vi "String_Find Any Expresion.vi"(5 "Multiline? (F)":bool, 7 "Ignore Case? (F)":bool, 8 "Error":errorcluster, 9 "Match Strings":string[](array[string]), 10 "Offset (0)":i32, 11 "String":string) -> (0 "Error Out":errorcluster, 1 "After Match Out":string, 2 "Whole Match Out":string, 3 "Before Match Out":string, 4 "Offset Past Match Out":i32)   [LabVIEW 2015]
uses:
  <vilib>/regexp/Match Regular Expression.xnode
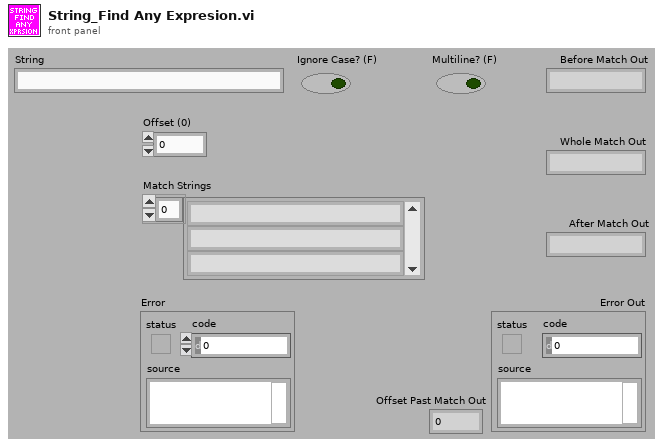
[diagram p1: front panel]
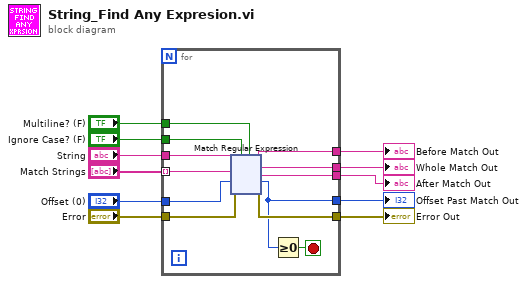
[diagram p0: block diagram]
diagram:
  n1 = for {
    tunnel: "String" -> [w12]
    tunnel: [w23] -> w10
    tunnel: [w22] -> w9
    tunnel: [w21] -> w8
    tunnel: [w15] -> w7
    tunnel: "Offset (0)" -> [w20]
    tunnel: "Error" -> [w19]
    tunnel: [w18] -> w4
    tunnel: "Ignore Case? (F)" -> [w17]
    tunnel: "Multiline? (F)" -> [w16]
    tunnel: "Match Strings" -> [w13] mode=indexing
    stop <- w14 stop-if-true
    n2 = xnode "Match Regular Expression"("input string"=w12, "regular expression"=w13, "offset (0)"=w20, "error in"=w19, "ignore case? (F)"=w17, "multiline? (F)"=w16) -> ("before match"=w23:string, "whole match"=w22:string, "after match"=w21:string, "offset past match"=w15:i32, "error out"=w18:errorcluster)
    n3 = Greater Or Equal To 0?(x=w15) -> (x >= 0?=w14:bool)
  }
  "Before Match Out" <- w10
  "Whole Match Out" <- w9
  "After Match Out" <- w8
  "Offset Past Match Out" <- w7
  "Error Out" <- w4
